vi "ShowTask(Sub).vi"(8 "error in (no error)":errorcluster, 10 "Message Enqueuer":refnum<class "Message Enqueuer.lvclass">, 11 "DAQ_Module in":refnum<class "DAQ_Module.lvclass">) -> (0 "error out":errorcluster, 3 "DAQ_Module out":refnum<class "DAQ_Module.lvclass">)   [LabVIEW 2025, in "DAQ_Module.lvlib" / "DAQ_Module.lvclass"]
uses:
  DAQ_Module.lvclass
  <vilib>/ActorFramework/Message Enqueuer/Message Enqueuer.lvclass
  DAQ_Abstr/Task_Abstr/Task_Abstr Messages/ShowPanel Msg/ShowPanel Msg.lvclass/ShowPanel Msg.ctl
  <vilib>/ActorFramework/Message Enqueuer/Message Enqueuer.lvclass/Message Enqueuer.ctl
  <vilib>/ActorFramework/Message Enqueuer/Enqueue.vi
  DAQ_Abstr/Task_Abstr/Task_Abstr Messages/ShowPanel Msg/ShowPanel Msg.lvclass
  <vilib>/ActorFramework/Message Priority Queue/Priority Enqueue.vi
  <vilib>/Test Bench Framework/Client Message(Context).vi
  DAQ_Module.lvclass/DAQ_Module.ctl
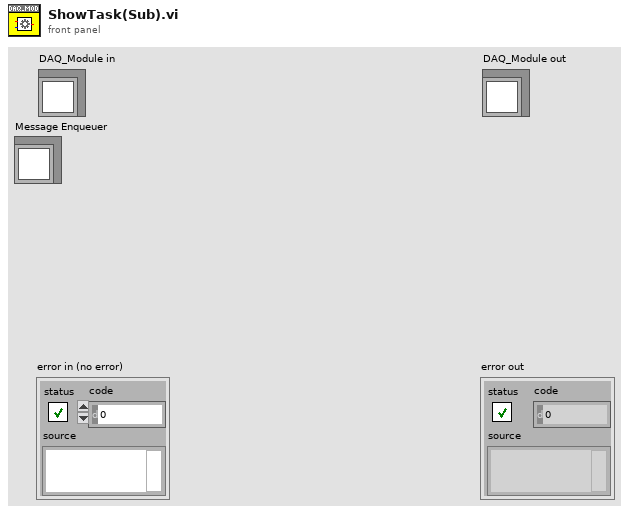
[diagram p1: front panel]
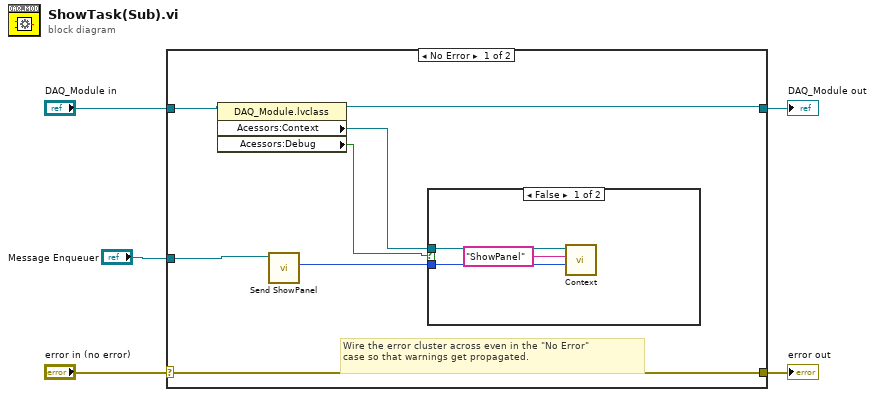
[diagram p0: block diagram]
diagram:
  n1 = case shown="No Error" "error in (no error)" {
    selector: "error in (no error)" -> [w12 w17]
    tunnel: [w12 w17] -> w4
    tunnel: [w9 w16] -> w2
    tunnel: "DAQ_Module in" -> [w10 w16]
    tunnel: "Message Enqueuer" -> [w7 _]
    frame No Error {
      # "Wire the error cluster across even in the \"No Error\"\ncase so that warnings get propagated."
      n2 = property class="DAQ_Module.lvclass"(reference=w10) -> (reference out=w9:refnum<class "DAQ_Module.lvclass">, "Acessors:Context"=w11:refnum<vi>, "Acessors:Debug"=w6:bool)  [unwired: 1 in, 1 out]
      n3 = call "Send ShowPanel.vi"("Message Enqueuer"=w7) -> ("FP.NativeWindow"=w8:u64)  [unwired: 8 in, 2 out]
      n4 = case shown="False" w6 {
        tunnel: w11 -> [w15 _]
        tunnel: w8 -> [w14 _]
        frame False {
          n5 = call-poly <vilib>:"Context.vi"("Value"=w14, "Msg"="ShowPanel", "Context"=w15) -> ()  [unwired: 8 in, 1 out]
        }
        frame True {
        }
      }
    }
    frame Error {
    }
  }
  "error out" <- w4
  "DAQ_Module out" <- w2
